vi "aotf_waveform.vi"(9 "Sweep Interval (µS)":u32, 10 "Actual Sweep Time (µS)":u32, 11 "Phase Shift (µS)":i32) -> (2 "Digital Waveform Graph":digitalwaveform(graph))   [LabVIEW 2013]
uses:
  <vilib>/Waveform/DWDTOps.llb/Digital Pattern Generator (Single Value).vi
  <vilib>/Waveform/DWDTOps.llb/DWDT Append Digital Samples.vi
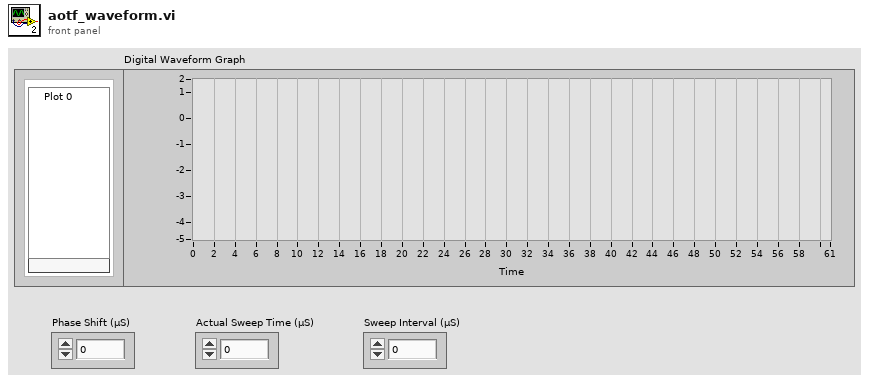
[diagram p1: front panel]
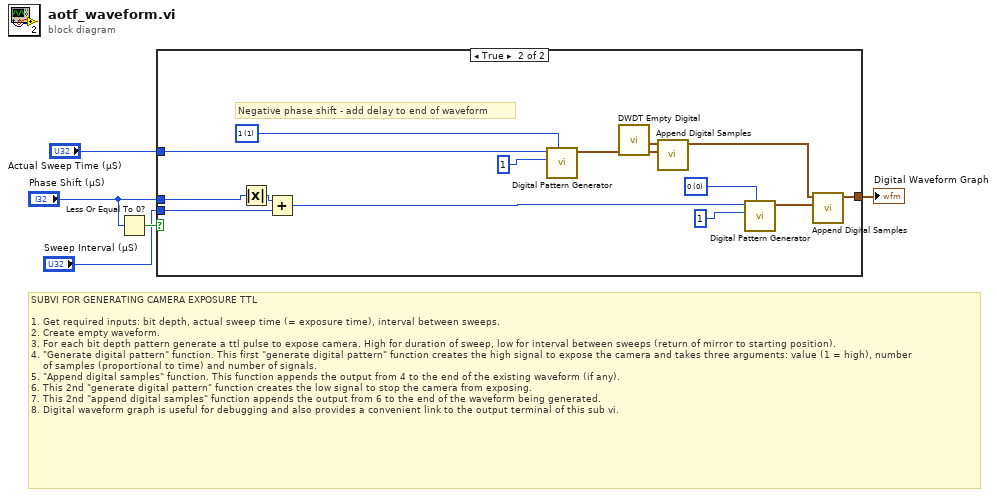
[diagram p0: block diagram]
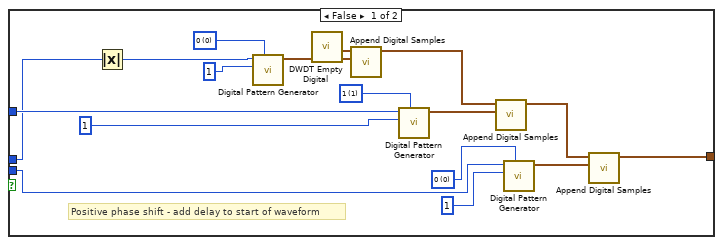
[diagram p2: hidden frame]
diagram:
  # "SUBVI FOR GENERATING CAMERA EXPOSURE TTL\n\n1. Get required inputs: bit depth, actual sweep time (= exposure time), interval between sweeps.\n2. Create empty waveform.\n3. For each bit depth pattern generate a ttl pulse to expose camera. High for duration of sweep, low for interval between sweeps (return of mirror to starting position).\n4. \"Generate digital pattern\" function. This first \"generate digital pattern\" function creates the high signal to expose the camera and takes three arguments: value (1 = high), number \n    of samples (proportional to time) and number of signals.\n5. \"Append digital samples\" function. This function appends the output from 4 to the end of the existing waveform (if any).\n6. This 2nd \"generate digital pattern\" function creates the low signal to stop the camera from exposing.\n7. This 2nd \"append digital samples\" function appends the output from 6 to the end of the waveform being generated.\n8. Digital waveform graph is useful for debugging and also provides a convenient link to the output terminal of this sub vi."
  n1 = Less Or Equal To 0?(x="Phase Shift (µS)") -> (x <= 0?=w5:bool)
  n2 = case shown="True" w5 {
    tunnel: "Phase Shift (µS)" -> [w7 w23]
    tunnel: "Actual Sweep Time (µS)" -> [w10 w28]
    tunnel: "Sweep Interval (µS)" -> [w9 w27]
    tunnel: [w8 w25] -> w1
    frame False {
      w13 = u8 0 items=["0", "1", "Z", "L", "H", "X", "T", "V"] ("value")
      w16 = u8 1 items=["0", "1", "Z", "L", "H", "X", "T", "V"] ("value")
      w19 = u8 0 items=["0", "1", "Z", "L", "H", "X", "T", "V"] ("value")
      # "Positive phase shift - add delay to start of waveform"
      n3 = Absolute Value(x=w7) -> (abs(x)=w6:i32)
      n4 = call-poly <vilib>:"Digital Pattern Generator.vi"("value"=w19, "number of signals"=u32 1, "number of samples"=w6) -> ("digital waveform"=w21:digitalwaveform)  [unwired: 7 in, 1 out]
      n5 = call <vilib>:"DWDT Empty Digital.vi"() -> ("digital waveform out"=w22:digitalwaveform)  [unwired: 5 in]
      n6 = call-poly <vilib>:"Append Digital Samples.vi"("digital waveform B"=w21, "digital waveform A"=w22) -> ("digital waveform out"=w20:digitalwaveform)  [unwired: 8 in, 1 out]
      n7 = call-poly <vilib>:"Digital Pattern Generator.vi"("value"=w16, "number of signals"=u32 1, "number of samples"=w10) -> ("digital waveform"=w17:digitalwaveform)  [unwired: 7 in, 1 out]
      n8 = call-poly <vilib>:"Append Digital Samples.vi"("digital waveform B"=w17, "digital waveform A"=w20) -> ("digital waveform out"=w11:digitalwaveform)  [unwired: 8 in, 1 out]
      n9 = call-poly <vilib>:"Digital Pattern Generator.vi"("value"=w13, "number of signals"=u32 1, "number of samples"=w9) -> ("digital waveform"=w14:digitalwaveform)  [unwired: 7 in, 1 out]
      n10 = call-poly <vilib>:"Append Digital Samples.vi"("digital waveform B"=w14, "digital waveform A"=w11) -> ("digital waveform out"=w8:digitalwaveform)  [unwired: 8 in, 1 out]
    }
    frame True {
      w30 = u8 0 items=["0", "1", "Z", "L", "H", "X", "T", "V"] ("value")
      w33 = u8 1 items=["0", "1", "Z", "L", "H", "X", "T", "V"] ("value")
      # "Negative phase shift - add delay to end of waveform"
      n11 = Absolute Value(x=w23) -> (abs(x)=w24:i32)
      n12 = Add(x=w24, y=w27) -> (x+y=w26:u32)
      n13 = call-poly <vilib>:"Digital Pattern Generator.vi"("value"=w33, "number of signals"=u32 1, "number of samples"=w28) -> ("digital waveform"=w35:digitalwaveform)  [unwired: 7 in, 1 out]
      n14 = call <vilib>:"DWDT Empty Digital.vi"() -> ("digital waveform out"=w36:digitalwaveform)  [unwired: 5 in]
      n15 = call-poly <vilib>:"Append Digital Samples.vi"("digital waveform B"=w35, "digital waveform A"=w36) -> ("digital waveform out"=w34:digitalwaveform)  [unwired: 8 in, 1 out]
      n16 = call-poly <vilib>:"Digital Pattern Generator.vi"("value"=w30, "number of signals"=u32 1, "number of samples"=w26) -> ("digital waveform"=w31:digitalwaveform)  [unwired: 7 in, 1 out]
      n17 = call-poly <vilib>:"Append Digital Samples.vi"("digital waveform B"=w31, "digital waveform A"=w34) -> ("digital waveform out"=w25:digitalwaveform)  [unwired: 8 in, 1 out]
    }
  }
  "Digital Waveform Graph" <- w1
